vi "Init Message Transport Notifier.vi"(8 "error in (no error)":errorcluster, 11 "Message":refnum<class "Message Interface.lvclass">) -> (0 "error out":errorcluster, 3 "Message Transport Notifier out":refnum<class "Message Transport Notifier.lvclass">)   [LabVIEW 2016, in "Stream Mediator.lvlib" / "Message Transport Notifier.lvclass"]
doc: "--\nCopyright © 2017 Composed SystemsI All rights reserved.\n\nAuthor: Jon McBee <jon.mcbee@composed.io>\n\nThis library is provided \"AS IS\" ,WITHOUT WARRANTIES OR\nCONDITIONS OF ANY KIND, either express or implied.\n\nComposed Systems -- composed.io\n\nStream 0.0.1.1\nJon McBee - Composed Systems\nCopyright (c) 2017, Composed Systems"
uses:
  <userlib>/Composed Systems/Stream/Mediator/Classes/Message Transport Notifier/Message Transport Notifier.lvclass
  <userlib>/Composed Systems/Stream/Mediator/Classes/Message Interface/Message Interface.lvclass
  <userlib>/Composed Systems/Stream/Mediator/Classes/Message Transport Notifier/Message Transport Notifier.lvclass/Message Transport Notifier.ctl
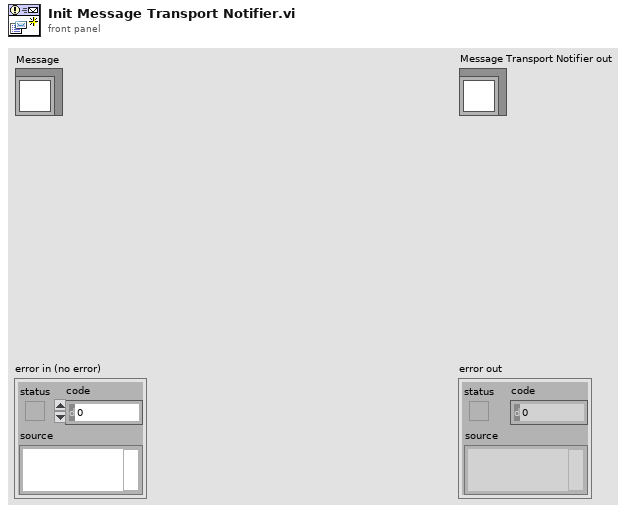
[diagram p1: front panel]
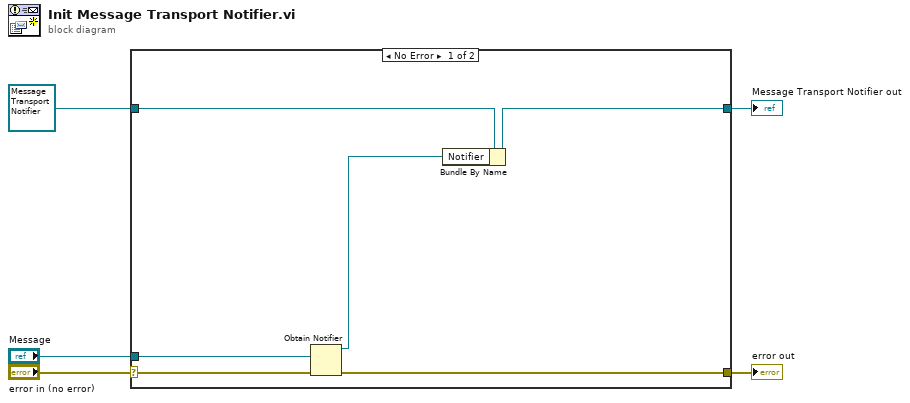
[diagram p0: block diagram]
diagram:
  n1 = case shown="No Error" "error in (no error)" {
    selector: "error in (no error)" -> [w9 w13]
    tunnel: [w8 w13] -> w4
    tunnel: [w10 w12] -> w2
    tunnel: refnum<class "Message Transport Notifier.lvclass"> refnum ("Message Transport Notifier in") -> [w11 w12]
    tunnel: "Message" -> [w6 _]
    frame No Error {
      n2 = Obtain Notifier(notification data type=w6, error in (no error)=w9) -> (notifier out=w7:refnum<notifier>, error out=w8:errorcluster)  [unwired: 2 in, 1 out]
      n3 = Bundle By Name(cluster=w11, "Notifier"=w7) -> (w10:refnum<class "Message Transport Notifier.lvclass">)
    }
    frame Error {
    }
  }
  "error out" <- w4
  "Message Transport Notifier out" <- w2
